vi "Array Of Clusters - Write Age.vi"(8 "error in (no error)":errorcluster, 11 "input array":T1(array[cluster])) -> (0 "error out":errorcluster, 3 "output array":T1(array[cluster]))   [LabVIEW 2013]
uses:
  ClassDefinitions/SimpleClassWithProperties/myClass.lvclass
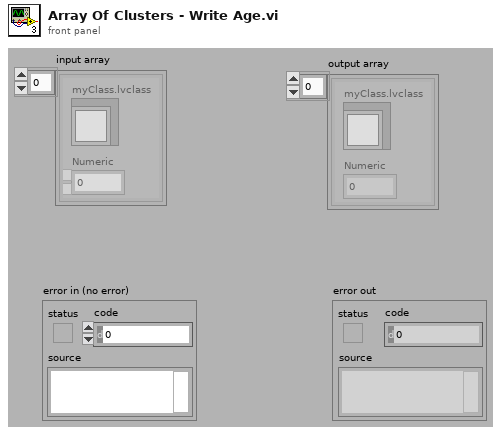
[diagram p1: front panel]
types:
  T1 = cluster{"myClass.lvclass":refnum<class "myClass.lvclass">, "Numeric":dbl}[]
  T2 = cluster{"myClass.lvclass":refnum<class "myClass.lvclass">, "Numeric":dbl}
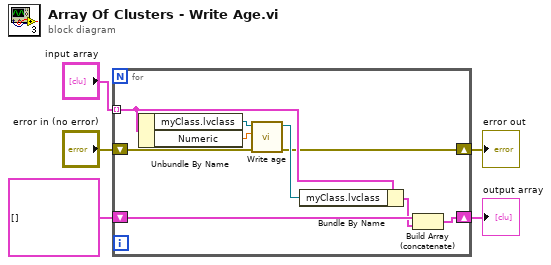
[diagram p0: block diagram]
diagram:
  n1 = for {
    tunnel: "input array" -> [w11] mode=indexing
    shift-right: [w8] -> w3
    shift-left: T1 [] ("input array") -> [w10]
    shift-right: [w6] -> w1
    shift-left: "error in (no error)" -> [w7]
    n2 = Unbundle By Name(w11) -> ("myClass.lvclass"=w13:refnum<class "myClass.lvclass">, "Numeric"=w14:dbl)
    n3 = call-dynamic "Write age.vi"("error in (no error)"=w7, "age"=w14, "myClass in"=w13) -> ("error out"=w6:errorcluster, "myClass out"=w12:refnum<class "myClass.lvclass">)  [unwired: 7 in]
    n4 = Bundle By Name(cluster=w11, "myClass.lvclass"=w12) -> (w9:T2)
    n5 = Build Array (concatenate)(w10, w9) -> (w8:T1)
  }
  "output array" <- w3
  "error out" <- w1
